vi "Read Voltage (List Current Sweep).vi"(5 "Delay Time (0.1 S)":dbl=0.1, 7 "Sweep Points (5)":i32=5, 8 "error in (no error)":errorcluster, 9 "Sweep List (A)":dbl[](array[numeric]), 10 "Source Measure Unit Channel (0: Channel A)":i32(ring) items=["Channel A", "Channel B"], 11 "VISA resource name":refnum<visa-resource-name>) -> (0 "error out":errorcluster, 2 "Voltage (V)":dbl[](array[numeric]), 3 "VISA resource name out":refnum<visa-resource-name>)   [LabVIEW 2019, in "Keithley 2600 Series.lvlib"]
doc: "Performs a current list sweep with voltage measured at every point."
uses:
  Keithley 2600 Series.lvlib
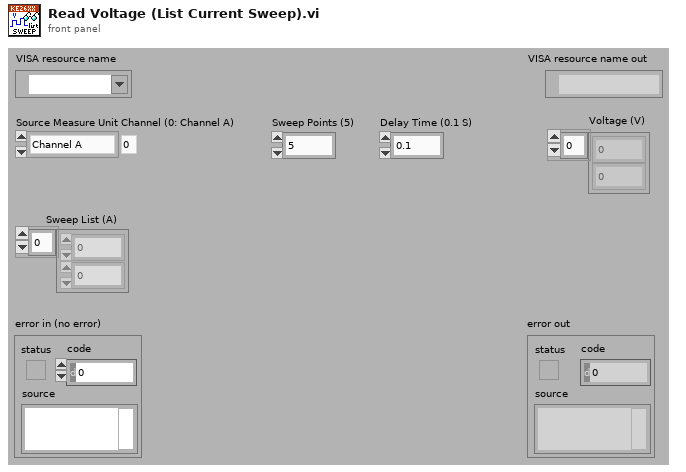
[diagram p1: front panel]
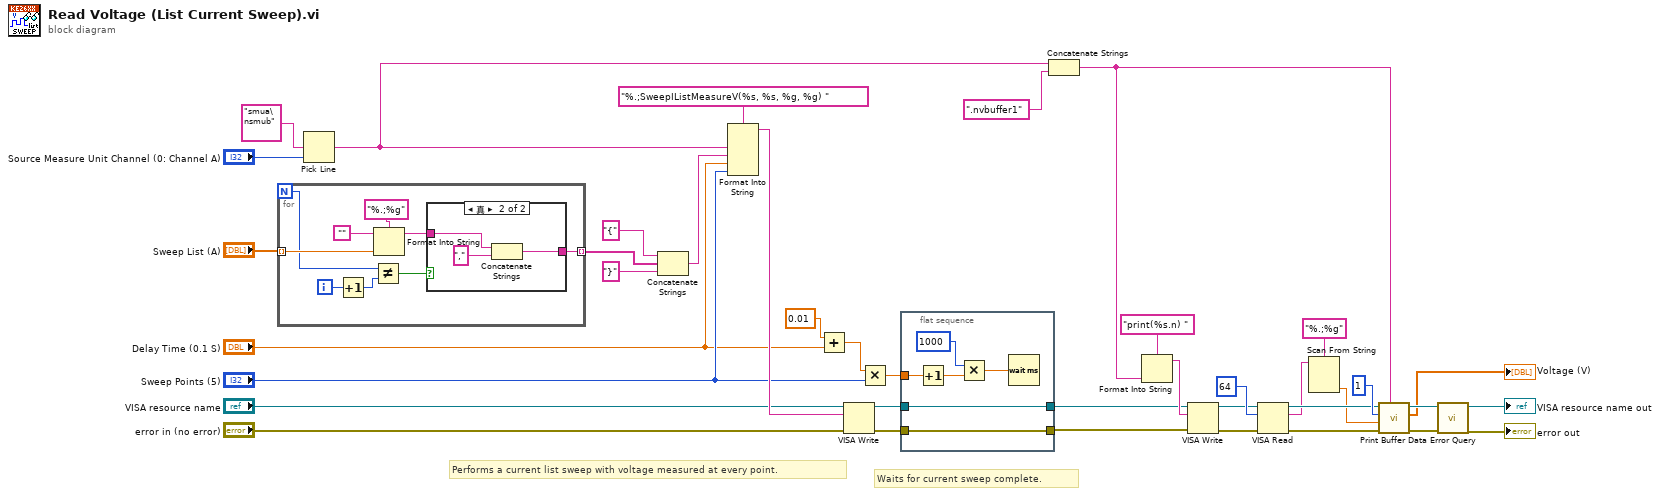
[diagram p0: block diagram]
diagram:
  # "Waits for current sweep complete."
  # "Performs a current list sweep with voltage measured at every point."
  n1 = for {
    N -> [w40]
    tunnel: "Sweep List (A)" -> [w48] mode=indexing
    tunnel: [w43] -> w31 mode=indexing
    i -> [w41]
    n2 = Increment(x=w41) -> (x+1=w42:i32)
    n3 = Not Equal?(x=w40, y=w42) -> (x != y?=w45:bool)
    n4 = Format Into String(format string="%.;%g", initial string="", w48) -> (resulting string=w44:string)  [unwired: 1 in, 1 out]
    n5 = case shown="真" w45 {
      tunnel: w44 -> [w49 w52]
      tunnel: [w49 w50] -> w43
      frame False {
      }
      frame True {
        n6 = Concatenate Strings(w52, ",") -> (w50:string)
      }
    }
  }
  n7 = Pick Line(multi-line string="smua\nsmub", line index="Source Measure Unit Channel (0: Channel A)") -> (output string=w3:string)  [unwired: 1 in]
  n8 = Concatenate Strings("{" ("string"), w31, "}") -> (w28:string)
  n9 = Format Into String(format string="%.;SweepIListMeasureV(%s, %s, %g, %g) ", w3, w28, "Delay Time (0.1 S)", "Sweep Points (5)") -> (resulting string=w38:string)  [unwired: 2 in, 1 out]
  n10 = Add(x=0.01, y="Delay Time (0.1 S)") -> (x+y=w22:dbl)
  n11 = VISA Write(VISA resource name="VISA resource name", write buffer=w38, error in (no error)="error in (no error)") -> (VISA resource name out=w26:refnum<visa-resource-name>, error out=w25:errorcluster)  [unwired: 1 out]
  n12 = Multiply(x=w22, y="Sweep Points (5)") -> (x*y=w21:dbl)
  n13 = flat-sequence {
    tunnel: w26 -> [w58]
    tunnel: w25 -> [w53]
    tunnel: [w58] -> w7
    tunnel: w21 -> [w56]
    tunnel: [w53] -> w6
    frame #0 {
      n14 = Increment(x=w56) -> (x+1=w55:dbl)
      n15 = Multiply(x=1000, y=w55) -> (x*y=w54:dbl)
      n16 = Wait (ms)(milliseconds to wait=w54) -> ()  [unwired: 1 out]
    }
  }
  n17 = Concatenate Strings(w3, ".nvbuffer1" ("string")) -> (w8:string)
  n18 = Format Into String(format string="print(%s.n) ", w8) -> (resulting string=w10:string)  [unwired: 2 in, 1 out]
  n19 = VISA Write(VISA resource name=w7, write buffer=w10, error in (no error)=w6) -> (VISA resource name out=w13:refnum<visa-resource-name>, error out=w12:errorcluster)  [unwired: 1 out]
  n20 = VISA Read(VISA resource name=w13, byte count=u32 64, error in (no error)=w12) -> (VISA resource name out=w18:refnum<visa-resource-name>, read buffer=w16:string, error out=w17:errorcluster)  [unwired: 1 out]
  n21 = Scan From String(format string="%.;%g", input string=w16) -> (output 1=w15:dbl)  [unwired: 3 in, 3 out]
  n22 = call "Print Buffer Data.vi"("Reading Buffer (smua.nvbuffer1)"=w8, "error in (no error)"=w17, "End Index (1)"=w15, "Start Index (1)"=1 ("Start Index (0)"), "VISA resource name"=w18) -> ("error out"=w4:errorcluster, "Buffer Data"=→"Voltage (V)":dbl[], "VISA resource name out"=w5:refnum<visa-resource-name>)  [unwired: 4 in]
  n23 = call "Error Query.vi"("error in (no error)"=w4, "VISA resource name"=w5) -> ("error out"=→"error out":errorcluster, "VISA resource name out"=→"VISA resource name out":refnum<visa-resource-name>)  [unwired: 6 in, 2 out]
